vi "Write Voltage.vi"(8 "error in (no error)":errorcluster, 10 "Voltage":dbl, 11 "Power Meter Display in":refnum<class "Power Meter Display.lvclass">) -> (0 "error out":errorcluster, 3 "Power Meter Display out":refnum<class "Power Meter Display.lvclass">)   [LabVIEW 2013, in "Display Panel.lvlib" / "Power Meter Display.lvclass"]
uses:
  Power Meter Display.lvclass
  Power Meter Display.lvclass/Power Meter Display.ctl
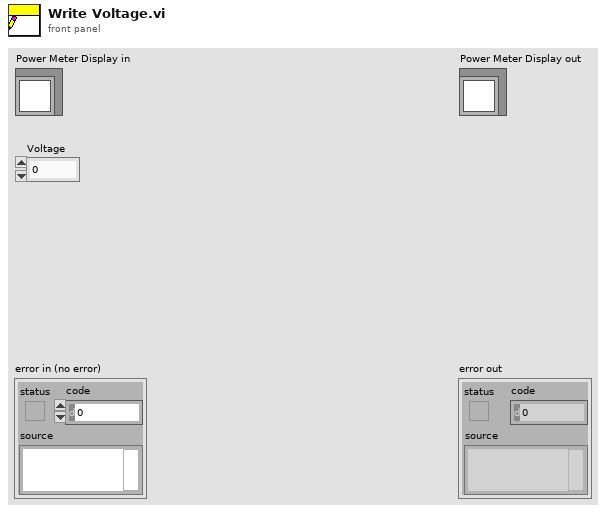
[diagram p1: front panel]
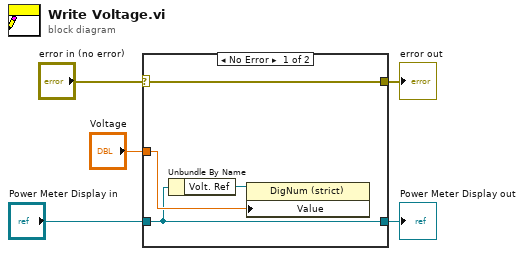
[diagram p0: block diagram]
diagram:
  n1 = case shown="No Error" "error in (no error)" {
    selector: "error in (no error)" -> [w9 w10]
    tunnel: [w9 w10] -> w4
    tunnel: [w6 w11] -> w2
    tunnel: "Power Meter Display in" -> [w6 w11]
    tunnel: "Voltage" -> [w7 _]
    frame No Error {
      n2 = Unbundle By Name(w6) -> ("Volt. Ref"=w8:refnum<vi>)
      n3 = property class="DigNum (strict)"(reference=w8, "Value"=w7) -> ()  [unwired: 1 in, 2 out]
    }
    frame Error {
    }
  }
  "error out" <- w4
  "Power Meter Display out" <- w2
